vi "Initialize Instrument.vi"(8 "error in (no error)":errorcluster, 10 "Reset":bool, 11 "VNA-Keysight PNA in":refnum<class "VNA-Keysight PNA.lvclass">) -> (0 "error out":errorcluster, 3 "VNA-Keysight PNA out":refnum<class "VNA-Keysight PNA.lvclass">)   [LabVIEW 2020, in "VNA-Keysight PNA.lvclass"]
uses:
  VNA-Keysight PNA.lvclass
  C:/Sandbox/RF Bench/Source Code/WiSpry Test Framework/Instruments/Instrument.lvclass
  C:/Sandbox/RF Bench/Source Code/WiSpry Test Framework/Instruments/Vector Network Analyzer/Vector Network Analyzer.lvclass
  <vilib>/Instr/_visa.llb/VISA Open Access Mode.ctl
  Instrument.lvclass/Instrument.ctl
  Vector Network Analyzer.lvclass/Vector Network Analyzer.ctl
  Instrument.lvclass
  Vector Network Analyzer.lvclass
  <instrlib>/Keysight PNA Series/Keysight PNA Series.lvlib
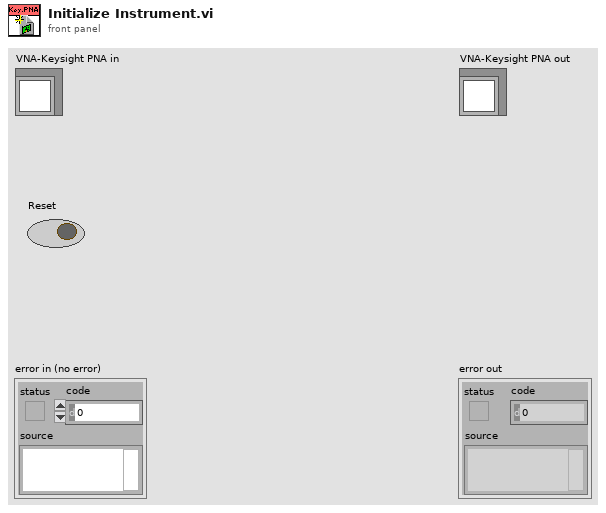
[diagram p1: front panel]
types:
  T1 = typedef "VISA Open Access Mode.ctl" = u32
  T2 = typedef "Instrument.lvclass/Interface String Cluster.ctl" = cluster{"Interface":string, "IDN string":string, "Instance":i32}
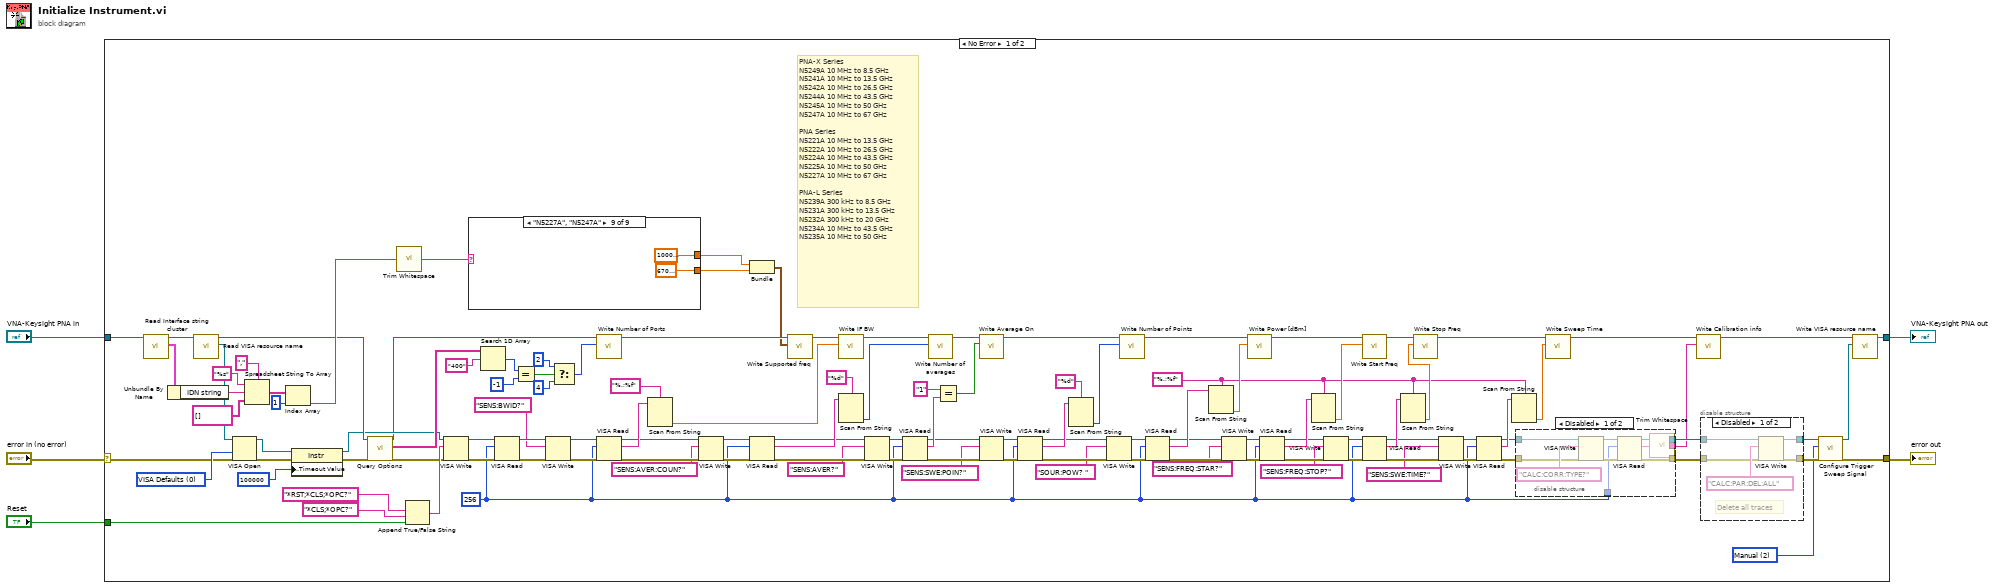
[diagram p0: block diagram]
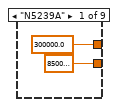
[diagram p4: hidden frame]
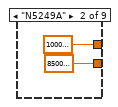
[diagram p5: hidden frame]
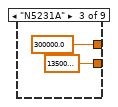
[diagram p6: hidden frame]
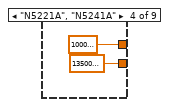
[diagram p7: hidden frame]
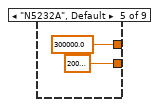
[diagram p8: hidden frame]
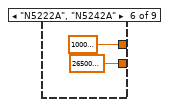
[diagram p9: hidden frame]
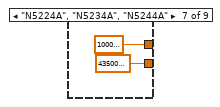
[diagram p10: hidden frame]
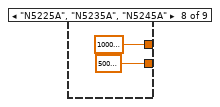
[diagram p11: hidden frame]
diagram:
  n1 = case shown="No Error" "error in (no error)" {
    selector: "error in (no error)" -> [w32 w166]
    tunnel: "VNA-Keysight PNA in" -> [w23 w167]
    tunnel: [w36 w166] -> w4
    tunnel: [w102 w167] -> w5
    tunnel: "Reset" -> [w47 _]
    frame No Error {
      w34 = 2 items=["Immediate", "External", "Manual"] ("Trigger Source (0: Immediate)")
      w49 = "%.;%f" ("format string")
      w11 = u32 256 ("byte count")
      w127 = T1 0 items=["VISA Defaults"=0, "Exclusive Lock"=1, "Load Configured Settings"=4] ("Access Mode")
      # "PNA-X Series\nN5249A 10 MHz to 8.5 GHz\nN5241A 10 MHz to 13.5 GHz\nN5242A 10 MHz to 26.5 GHz\nN5244A 10 MHz to 43.5 GHz\nN5245A 10 MHz to 50 GHz\nN5247A 10 MHz to 67 GHz\n\nPNA Series\nN5221A 10 MHz to 13.5 GHz\nN5222A 10 MHz to 26.5 GHz\nN5224A 10 MHz to 43.5 GHz\nN5225A 10 MHz to 50 GHz\nN5227A 10 MHz to 67 GHz\n\nPNA-L Series\nN5239A 300 kHz to 8.5 GHz\nN5231A 300 kHz to 13.5 GHz\nN5232A 300 kHz to 20 GHz\nN5234A 10 MHz to 43.5 GHz\nN5235A 10 MHz to 50 GHz"
      n2 = call "Read Interface string cluster.vi"("Instrument in"=w23) -> ("Interface sting cluster"=w21:T2, "Instrument out"=w22:refnum<class "VNA-Keysight PNA.lvclass">)  [unwired: 9 in]
      n3 = Unbundle By Name(w21) -> ("IDN string"=w27:string)
      n4 = call "Read VISA resource name.vi"("Instrument in"=w22) -> ("VISA resource name"=w128:refnum<visa-resource-name>, "Instrument out"=w9:refnum<class "VNA-Keysight PNA.lvclass">)  [unwired: 9 in]
      n5 = VISA Open(access mode=w127, error in (no error)=w32, VISA resource name=w128) -> (VISA resource name=w125:refnum<visa-resource-name>, error out=w33:errorcluster)  [unwired: 2 in]
      n6 = Spreadsheet String To Array(delimiter (Tab)=",", format string="%s", spreadsheet string=w27, array type (2D Dbl)=string[] []) -> (array=w28:string[])
      n7 = Index Array(array=w28, index=1) -> (element=w24:string)
      n8 = property class="Instr"(reference=w125, error in=w33, "General Settings:Timeout Value"=u32 100000) -> (reference out=w7:refnum<visa-resource-name>, error out=w8:errorcluster)
      n9 = call-dynamic "Query Options.vi"("error in (no error)"=w8, "Instrument in"=w9) -> ("error out"=w31:errorcluster, "Options"=w46:string[], "Instrument out"=w6:refnum<class "VNA-Keysight PNA.lvclass">)  [unwired: 7 in]
      n10 = call <vilib>:"Trim Whitespace.vi"("string"=w24) -> ("trimmed string"=w20:string)  [unwired: 1 in]
      n11 = Append True/False String(1:w47, 2:"*CLS;*OPC?" ("false string"), 3:"*RST;*CLS;*OPC?" ("Default Setup String")) -> (0:w122:string)  [unwired: 1 in]
      n12 = VISA Write(VISA resource name=w7, write buffer=w122, error in (no error)=w31) -> (VISA resource name out=w120:refnum<visa-resource-name>, error out=w121:errorcluster)  [unwired: 1 out]
      n13 = case shown="\"N5227A\", \"N5247A\"" w20 {
        tunnel: [8500000000.0 8500000000.0 13500000000.0 13500000000.0 20000000000.0 26500000000.0 43500000000.0 50000000000.0 67000000000.0] -> w19
        tunnel: [300000.0 10000000.0 300000.0 10000000.0 300000.0 10000000.0 10000000.0 10000000.0 10000000.0] -> w18
        frame "N5239A" {
        }
        frame "N5249A" {
        }
        frame "N5231A" {
        }
        frame "N5221A", "N5241A" {
        }
        frame "N5232A", Default {
        }
        frame "N5222A", "N5242A" {
        }
        frame "N5224A", "N5234A", "N5244A" {
        }
        frame "N5225A", "N5235A", "N5245A" {
        }
        frame "N5227A", "N5247A" {
        }
      }
      n14 = Search 1D Array(1D array=w46, element="400") -> (index of element=w44:i32)  [unwired: 1 in]
      n15 = VISA Read(VISA resource name=w120, byte count=w11, error in (no error)=w121) -> (VISA resource name out=w109:refnum<visa-resource-name>, error out=w110:errorcluster)  [unwired: 2 out]
      n16 = Equal?(x=w44, y=-1) -> (x = y?=w42:bool)
      n17 = VISA Write(VISA resource name=w109, write buffer="SENS:BWID?", error in (no error)=w110) -> (VISA resource name out=w111:refnum<visa-resource-name>, error out=w107:errorcluster)  [unwired: 1 out]
      n18 = Select(t=2 ("Number of Ports"), s=w42, f=4 ("Number of Ports")) -> (s? t:f=w39:i32)
      n19 = call "Write Number of Ports.vi"("Number of Ports"=w39, "Vector Network Analyzer in"=w6) -> ("Vector Network Analyzer out"=w119:refnum<class "VNA-Keysight PNA.lvclass">)  [unwired: 9 in]
      n20 = VISA Read(VISA resource name=w111, byte count=w11, error in (no error)=w107) -> (VISA resource name out=w100:refnum<visa-resource-name>, read buffer=w105:string, error out=w99:errorcluster)  [unwired: 1 out]
      n21 = Scan From String(format string="%.;%f", input string=w105) -> (output 1=w104:dbl)  [unwired: 3 in, 3 out]
      n22 = VISA Write(VISA resource name=w100, write buffer="SENS:AVER:COUN?", error in (no error)=w99) -> (VISA resource name out=w97:refnum<visa-resource-name>, error out=w101:errorcluster)  [unwired: 1 out]
      n23 = Bundle(w18, w19) -> (w118:cluster{dbl, dbl})  [unwired: 1 in]
      n24 = VISA Read(VISA resource name=w97, byte count=w11, error in (no error)=w101) -> (VISA resource name out=w91:refnum<visa-resource-name>, read buffer=w96:string, error out=w90:errorcluster)  [unwired: 1 out]
      n25 = call "Write Supported freq.vi"("Supported freq"=w118, "Vector Network Analyzer in"=w119) -> ("Vector Network Analyzer out"=w103:refnum<class "VNA-Keysight PNA.lvclass">)  [unwired: 9 in]
      n26 = call "Write IF BW.vi"("IF BW"=w104, "Vector Network Analyzer in"=w103) -> ("Vector Network Analyzer out"=w117:refnum<class "VNA-Keysight PNA.lvclass">)  [unwired: 9 in]
      n27 = Scan From String(format string="%d", input string=w96) -> (output 1=w94:i32)  [unwired: 3 in, 3 out]
      n28 = VISA Write(VISA resource name=w91, write buffer="SENS:AVER?", error in (no error)=w90) -> (VISA resource name out=w93:refnum<visa-resource-name>, error out=w92:errorcluster)  [unwired: 1 out]
      n29 = VISA Read(VISA resource name=w93, byte count=w11, error in (no error)=w92) -> (VISA resource name out=w83:refnum<visa-resource-name>, read buffer=w88:string, error out=w82:errorcluster)  [unwired: 1 out]
      n30 = call "Write Number of averages.vi"("Number of averages"=w94, "Vector Network Analyzer in"=w117) -> ("Vector Network Analyzer out"=w116:refnum<class "VNA-Keysight PNA.lvclass">)  [unwired: 9 in]
      n31 = Equal?(x="1", y=w88) -> (x = y?=w86:bool)
      n32 = call "Write Average On.vi"("Average On"=w86, "Vector Network Analyzer in"=w116) -> ("Vector Network Analyzer out"=w115:refnum<class "VNA-Keysight PNA.lvclass">)  [unwired: 9 in]
      n33 = VISA Write(VISA resource name=w83, write buffer="SENS:SWE:POIN?", error in (no error)=w82) -> (VISA resource name out=w84:refnum<visa-resource-name>, error out=w85:errorcluster)  [unwired: 1 out]
      n34 = VISA Read(VISA resource name=w84, byte count=w11, error in (no error)=w85) -> (VISA resource name out=w75:refnum<visa-resource-name>, read buffer=w79:string, error out=w74:errorcluster)  [unwired: 1 out]
      n35 = Scan From String(format string="%d", input string=w79) -> (output 1=w78:i32)  [unwired: 3 in, 3 out]
      n36 = VISA Write(VISA resource name=w75, write buffer="SOUR:POW? ", error in (no error)=w74) -> (VISA resource name out=w77:refnum<visa-resource-name>, error out=w76:errorcluster)  [unwired: 1 out]
      n37 = call "Write Number of Points.vi"("Number of Points"=w78, "Vector Network Analyzer in"=w115) -> ("Vector Network Analyzer out"=w114:refnum<class "VNA-Keysight PNA.lvclass">)  [unwired: 9 in]
      n38 = VISA Read(VISA resource name=w77, byte count=w11, error in (no error)=w76) -> (VISA resource name out=w68:refnum<visa-resource-name>, read buffer=w72:string, error out=w67:errorcluster)  [unwired: 1 out]
      n39 = Scan From String(format string=w49, input string=w72) -> (output 1=w71:dbl)  [unwired: 3 in, 3 out]
      n40 = VISA Write(VISA resource name=w68, write buffer="SENS:FREQ:STAR?", error in (no error)=w67) -> (VISA resource name out=w69:refnum<visa-resource-name>, error out=w70:errorcluster)  [unwired: 1 out]
      n41 = call "Write Power [dBm].vi"("Power [dBm]"=w71, "Vector Network Analyzer in"=w114) -> ("Vector Network Analyzer out"=w113:refnum<class "VNA-Keysight PNA.lvclass">)  [unwired: 9 in]
      n42 = VISA Read(VISA resource name=w69, byte count=w11, error in (no error)=w70) -> (VISA resource name out=w62:refnum<visa-resource-name>, read buffer=w65:string, error out=w61:errorcluster)  [unwired: 1 out]
      n43 = Scan From String(format string=w49, input string=w65) -> (output 1=w64:dbl)  [unwired: 3 in, 3 out]
      n44 = VISA Write(VISA resource name=w62, write buffer="SENS:FREQ:STOP?", error in (no error)=w61) -> (VISA resource name out=w63:refnum<visa-resource-name>, error out=w59:errorcluster)  [unwired: 1 out]
      n45 = call "Write Start Freq.vi"("Start Freq"=w64, "Vector Network Analyzer in"=w113) -> ("Vector Network Analyzer out"=w112:refnum<class "VNA-Keysight PNA.lvclass">)  [unwired: 9 in]
      n46 = VISA Read(VISA resource name=w63, byte count=w11, error in (no error)=w59) -> (VISA resource name out=w54:refnum<visa-resource-name>, read buffer=w57:string, error out=w53:errorcluster)  [unwired: 1 out]
      n47 = Scan From String(format string=w49, input string=w57) -> (output 1=w58:dbl)  [unwired: 3 in, 3 out]
      n48 = call "Write Stop Freq.vi"("Stop Freq"=w58, "Vector Network Analyzer in"=w112) -> ("Vector Network Analyzer out"=w51:refnum<class "VNA-Keysight PNA.lvclass">)  [unwired: 9 in]
      n49 = VISA Write(VISA resource name=w54, write buffer="SENS:SWE:TIME?", error in (no error)=w53) -> (VISA resource name out=w55:refnum<visa-resource-name>, error out=w56:errorcluster)  [unwired: 1 out]
      n50 = VISA Read(VISA resource name=w55, byte count=w11, error in (no error)=w56) -> (VISA resource name out=w14:refnum<visa-resource-name>, read buffer=w50:string, error out=w15:errorcluster)  [unwired: 1 out]
      n51 = Scan From String(format string=w49, input string=w50) -> (output 1=w48:dbl)  [unwired: 3 in, 3 out]
      n52 = disable-structure shown="Disabled" {
        disable-tunnel: w15 -> [w142 w146]
        disable-tunnel: w14 -> [w141 w147]
        disable-tunnel: [w140 w146] -> w13
        disable-tunnel: [w139 w147] -> w12
        disable-tunnel: w11 -> [w138 _]
        disable-tunnel: [w136 _] -> w10
        frame Disabled {
          n53 = VISA Write(VISA resource name=w141, write buffer="CALC:CORR:TYPE?", error in (no error)=w142) -> (VISA resource name out=w144:refnum<visa-resource-name>, error out=w143:errorcluster)  [unwired: 1 out]
          n54 = VISA Read(VISA resource name=w144, byte count=w138, error in (no error)=w143) -> (VISA resource name out=w139:refnum<visa-resource-name>, read buffer=w137:string, error out=w140:errorcluster)  [unwired: 1 out]
          n55 = call <vilib>:"Trim Whitespace.vi"("string"=w137) -> ("trimmed string"=w136:string)  [unwired: 1 in]
        }
        frame Enabled {
          # "Doesn't work with 1-port cal?"
        }
      }
      n56 = call "Write Sweep Time.vi"("Sweep Time"=w48, "Vector Network Analyzer in"=w51) -> ("Vector Network Analyzer out"=w17:refnum<class "VNA-Keysight PNA.lvclass">)  [unwired: 9 in]
      n57 = call-dynamic "Write Calibration info.vi"("Calibration info"=w10, "Vector Network Analyzer in"=w17) -> ("Vector Network Analyzer out"=w16:refnum<class "VNA-Keysight PNA.lvclass">)  [unwired: 9 in]
      n58 = disable-structure shown="Disabled" {
        disable-tunnel: [w132 w135] -> w38
        disable-tunnel: [w131 w134] -> w37
        disable-tunnel: w13 -> [w130 w134]
        disable-tunnel: w12 -> [w129 w135]
        frame Disabled {
          # "Delete all traces"
          n59 = VISA Write(VISA resource name=w129, write buffer="CALC:PAR:DEL:ALL", error in (no error)=w130) -> (VISA resource name out=w132:refnum<visa-resource-name>, error out=w131:errorcluster)  [unwired: 1 out]
        }
        frame Enabled {
        }
      }
      n60 = call <instrlib>:"Configure Trigger Sweep Signal.vi"("error in (no error)"=w37, "Trigger Source (0: Immediate)"=w34, "VISA resource name"=w38) -> ("error out"=w36:errorcluster, "VISA resource name out"=w35:refnum<visa-resource-name>)  [unwired: 7 in]
      n61 = call "Write VISA resource name.vi"("VISA resource name"=w35, "Instrument in"=w16) -> ("Instrument out"=w102:refnum<class "VNA-Keysight PNA.lvclass">)  [unwired: 9 in]
    }
    frame Error {
    }
  }
  "error out" <- w4
  "VNA-Keysight PNA out" <- w5
